vi "Merge_Raw_DF_metadata.vi"(4 "New Values In":string[](array[string]), 5 "New Chs In":string[](array[string]), 6 "Orig Values In":string[][](array[string]), 7 "Orig Chs In":string[](array[string])) -> (0 "Channel Values Out":string[][](array[string]), 1 "Ch names Out":string[](array[string]), 3 "Original values":string[](array[string]))   [LabVIEW 2020]
panel:
  out "Case":string
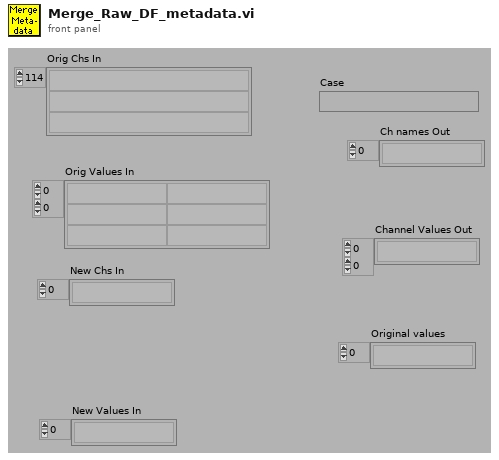
[diagram p1: front panel]
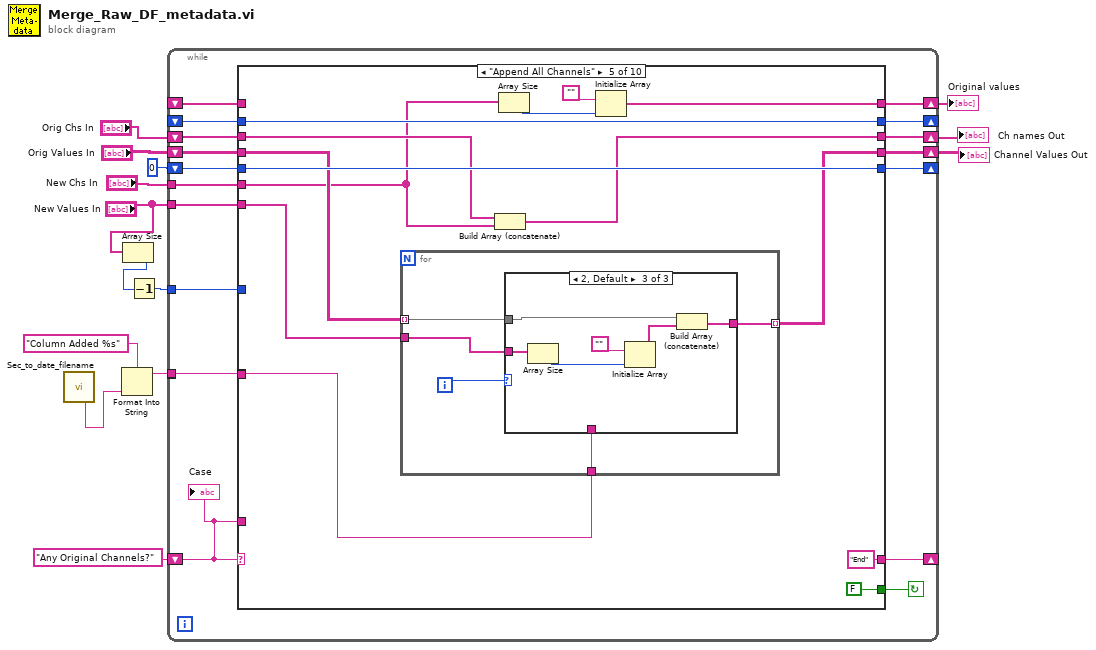
[diagram p0: block diagram]
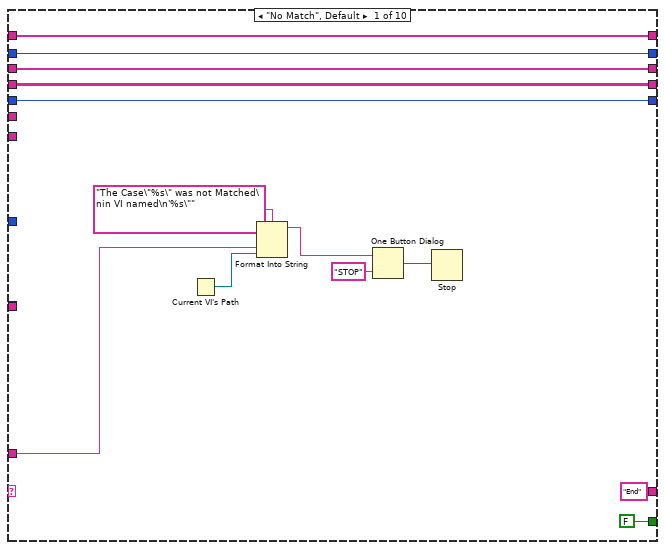
[diagram p2: hidden frame]
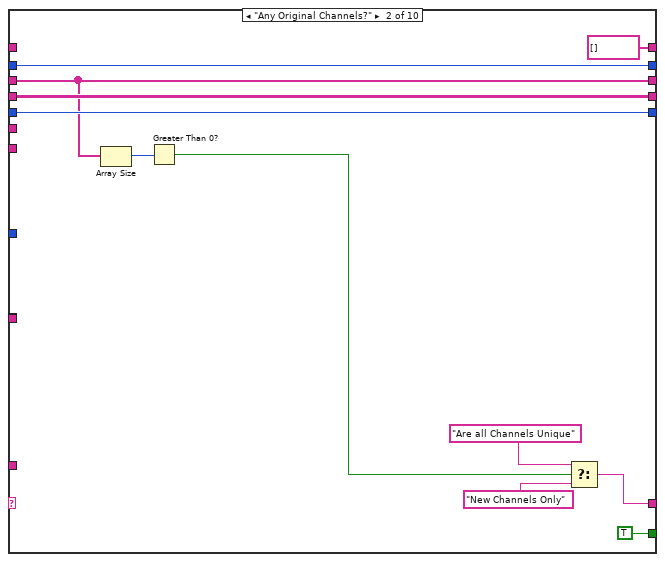
[diagram p3: hidden frame]
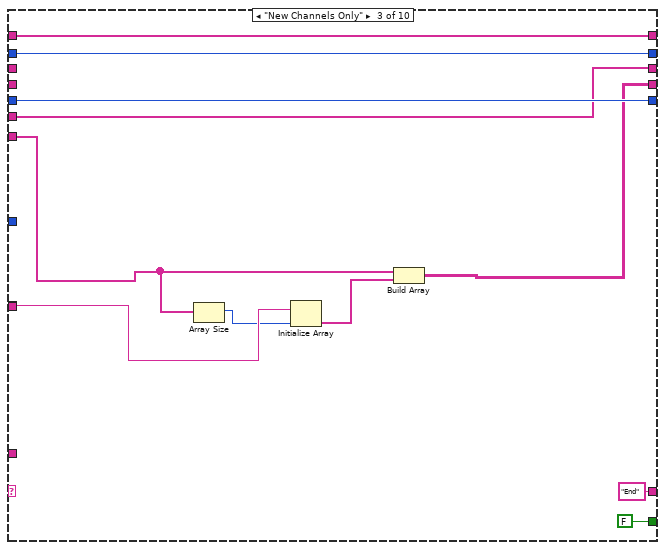
[diagram p4: hidden frame]
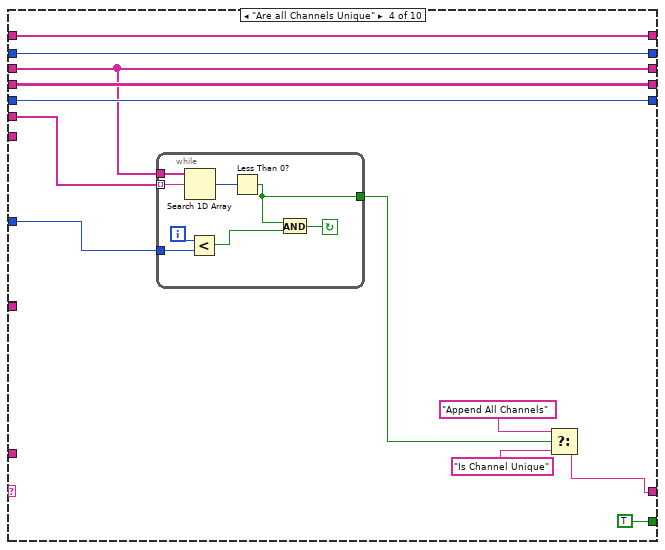
[diagram p5: hidden frame]
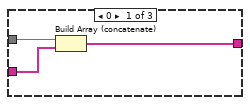
[diagram p6: hidden frame]
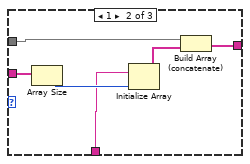
[diagram p7: hidden frame]
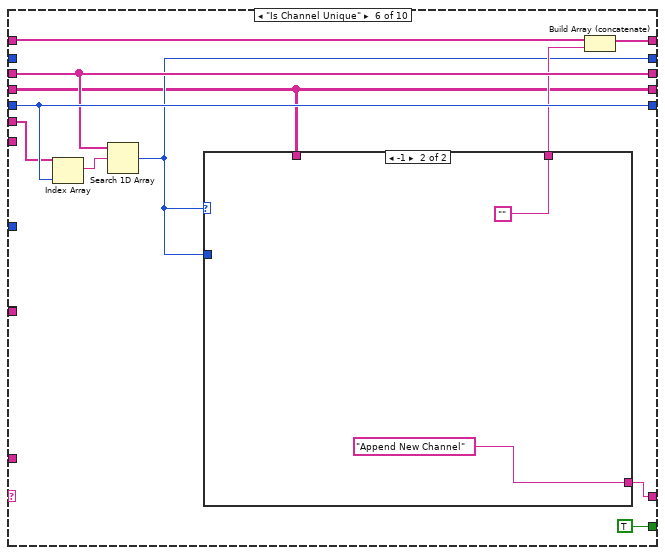
[diagram p8: hidden frame]
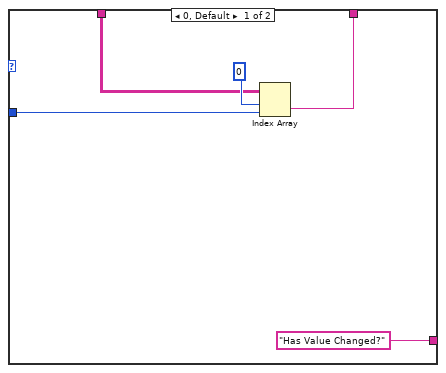
[diagram p9: hidden frame]
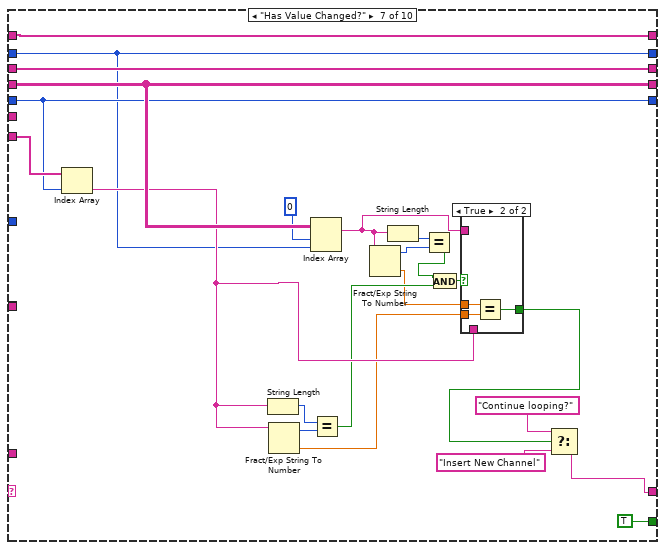
[diagram p10: hidden frame]
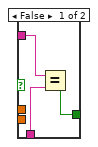
[diagram p11: hidden frame]
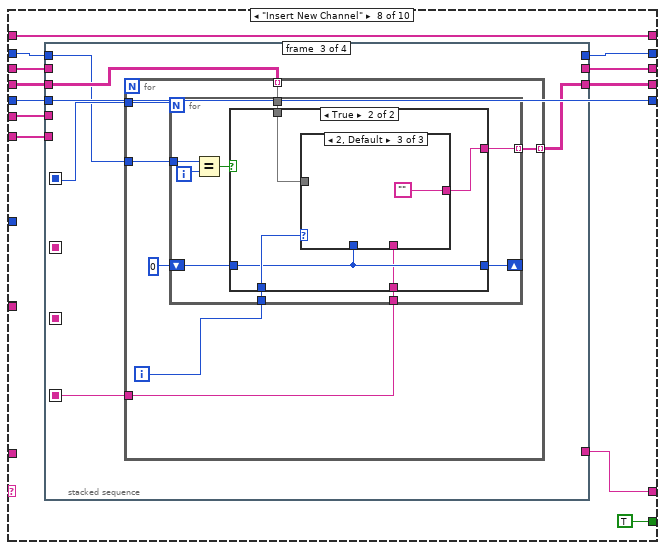
[diagram p12: hidden frame]
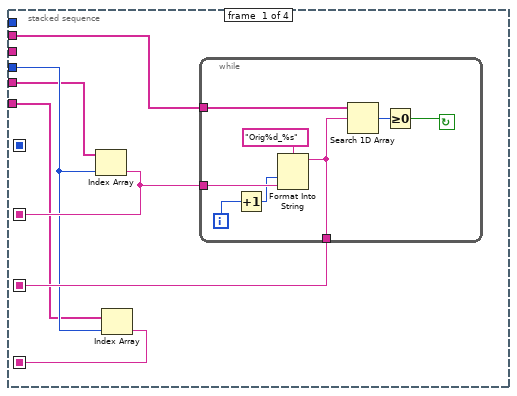
[diagram p13: hidden frame]
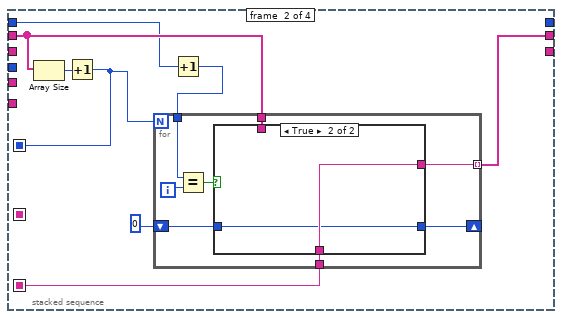
[diagram p14: hidden frame]
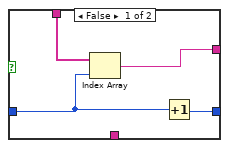
[diagram p15: hidden frame]
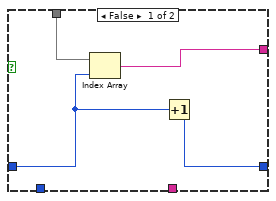
[diagram p16: hidden frame]
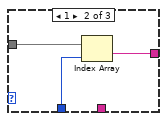
[diagram p18: hidden frame]
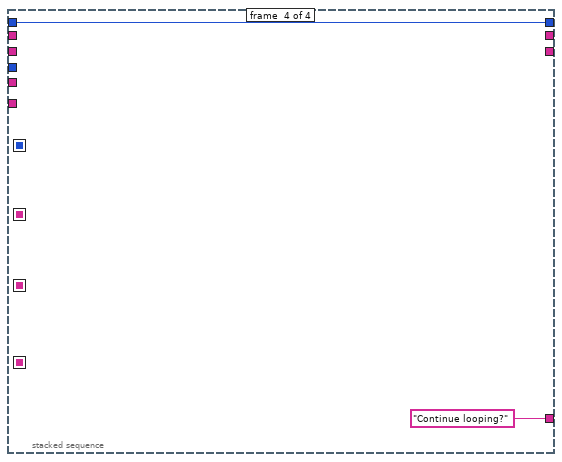
[diagram p19: hidden frame]
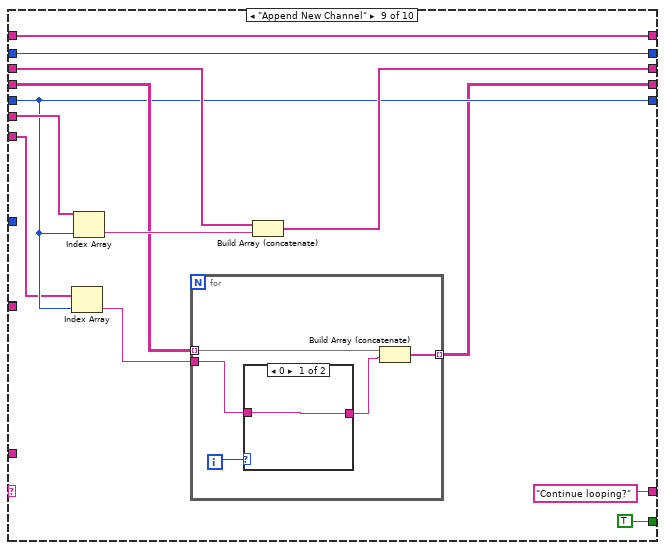
[diagram p20: hidden frame]
diagram:
  n1 = call "Sec_to_date_filename.vi"() -> ("YYYY-mm-DD HH:MM"=w1:string)  [unwired: 6 in, 9 out]
  n2 = Format Into String(format string="Column Added %s" ("Format String"), w1) -> (resulting string=w4:string)  [unwired: 2 in, 1 out]
  n3 = Array Size(array="New Values In") -> (size(s)=w10:i32)
  n4 = Decrement(x=w10) -> (x-1=w9:i32)
  n5 = while {
    tunnel: w4 -> [w17]
    tunnel: w4 -> [w18]
    shift-left: _ -> [w20]
    shift-right: [w19] -> _
    tunnel: "New Values In" -> [w21]
    tunnel: "New Chs In" -> [w22]
    tunnel: w9 -> [w23]
    shift-left: 0 -> [w24]
    shift-right: [w25] -> _
    shift-left: "Orig Values In" -> [w27]
    shift-right: [w26] -> w12
    shift-left: "Orig Chs In" -> [w28]
    shift-right: [w29] -> w13
    shift-left: "Any Original Channels?" -> [w31]
    shift-right: [w30] -> _
    shift-right: [w15] -> w2
    shift-left: _ -> [w16]
    stop <- w32 continue-if-true
    n6 = case shown="\"Append All Channels\"" w31 {
      tunnel: [FALSE ("Results File?") TRUE ("Results File?") FALSE ("Results File?") TRUE ("Results File?") FALSE ("Results File?") TRUE ("Results File?") TRUE ("Results File?") TRUE ("Results File?") TRUE ("Results File?") w280] -> w32
      tunnel: w31 -> [w40 _ _ _ _ _ _ _ _ _]
      tunnel: w22 -> [_ _ w62 w72 w89 w127 _ w177 w266 _]
      tunnel: w21 -> [_ _ w61 _ w95 _ w159 w176 w260 _]
      tunnel: ["End" w51 "End" ("f") w78 "End" ("f") w131 w160 w172 "Continue looping?" "Is Channel Unique"] -> w30
      tunnel: [w37 w49 w62 w73 w97 w128 w162 w173 w263 w282] -> w29
      tunnel: w28 -> [w37 w49 _ w73 w98 w128 w162 w179 w264 w282]
      tunnel: w27 -> [w36 w55 _ w77 w96 w122 w158 w174 w262 w283]
      tunnel: [w36 w55 w63 w77 w94 w122 w158 w175 w258 w283] -> w26
      tunnel: [w35 w54 w66 w76 w100 w130 w150 w178 w261 w277] -> w25
      tunnel: w24 -> [w35 w54 w66 w76 w100 w130 w150 w178 w261 w278]
      tunnel: w23 -> [_ _ _ w71 _ _ _ _ _ w281]
      tunnel: w20 -> [w34 w53 w65 w69 w93 _ w149 w171 w256 w276]
      tunnel: [w34 w53 w65 w69 w93 w123 w149 w170 w256 w276] -> w19
      tunnel: w18 -> [_ _ w60 _ w92 _ _ _ _ _]
      tunnel: w17 -> [_ _ _ _ _ _ _ _ _ _]
      tunnel: w16 -> [w33 _ w57 w68 _ w125 w140 w169 w255 w275]
      tunnel: [w33 string[] [] w57 w68 w88 w124 w140 w169 w255 w275] -> w15
      frame "No Match", Default {
        n7 = Current VI's Path() -> (path=w41:path)
        n8 = Format Into String(format string="The Case\"%s\" was not Matched\nin VI named\n'%s\"" ("Format String"), w40, w41) -> (resulting string=w44:string)  [unwired: 2 in, 1 out]
        n9 = One Button Dialog(message=w44, button name ("OK")="STOP") -> (true=w42:bool)
        n10 = Stop(stop? (T)=w42) -> ()
      }
      frame "Any Original Channels?" {
        n11 = Array Size(array=w49) -> (size(s)=w48:i32)
        n12 = Greater Than 0?(x=w48) -> (x > 0?=w47:bool)
        n13 = Select(t="Are all Channels Unique", s=w47, f="New Channels Only") -> (s? t:f=w51:string)
      }
      frame "New Channels Only" {
        n14 = Array Size(array=w61) -> (size(s)=w59:i32)
        n15 = Initialize Array(w60, w59) -> (w58:string[])
        n16 = Build Array(w61, w58) -> (w63:string[][])
      }
      frame "Are all Channels Unique" {
        n17 = while {
          tunnel: [w80] -> w70
          tunnel: w71 -> [w83]
          tunnel: w72 -> [w86] mode=indexing
          tunnel: w73 -> [w87]
          i -> [w84]
          stop <- w81 continue-if-true
          n18 = Search 1D Array(1D array=w87, element=w86) -> (index of element=w85:i32)  [unwired: 1 in]
          n19 = Less?(x=w84, y=w83) -> (x < y?=w82:bool)
          n20 = Less Than 0?(x=w85) -> (x < 0?=w80:bool)
          n21 = And(x=w80, y=w82) -> (x .and. y?=w81:bool)
        }
        n22 = Select(t="Append All Channels" ("f"), s=w70, f="Is Channel Unique") -> (s? t:f=w78:string)
      }
      frame "Append All Channels" {
        n23 = for {
          tunnel: w96 -> [w106] mode=indexing
          tunnel: w95 -> [w105]
          tunnel: [w104] -> w94 mode=indexing
          tunnel: w92 -> [w103]
          i -> [w102]
          n24 = case shown="2, Default" w102 {
            tunnel: w106 -> [w109 w111 w118]
            tunnel: w105 -> [w108 w115 w121]
            tunnel: [w107 w110 w117] -> w104
            tunnel: w103 -> [_ w113 _]
            frame 0 {
              n25 = Build Array (concatenate)(w109, w108) -> (w107:string[])
            }
            frame 1 {
              n26 = Array Size(array=w115) -> (size(s)=w114:i32)
              n27 = Initialize Array(w113, w114) -> (w112:string[])
              n28 = Build Array (concatenate)(w111, w112) -> (w110:string[])
            }
            frame 2, Default {
              n29 = Array Size(array=w121) -> (size(s)=w120:i32)
              n30 = Initialize Array("", w120) -> (w119:string[])
              n31 = Build Array (concatenate)(w118, w119) -> (w117:string[])
            }
          }
        }
        n32 = Build Array (concatenate)(w98, w89) -> (w97:string[])
        n33 = Array Size(array=w89) -> (size(s)=w90:i32)
        n34 = Initialize Array("", w90) -> (w88:string[])
      }
      frame "Is Channel Unique" {
        n35 = Index Array(array=w127, index=w130) -> (element=w129:string)
        n36 = Search 1D Array(1D array=w128, element=w129) -> (index of element=w123:i32)  [unwired: 1 in]
        n37 = case shown="-1" w123 {
          tunnel: ["Has Value Changed?" ("f") "Append New Channel"] -> w131
          tunnel: [w135 ""] -> w126
          tunnel: w123 -> [w136 _]
          tunnel: w122 -> [w134 _]
          frame 0, Default {
            n38 = Index Array(array=w134, index (row)=0, index (col)=w136) -> (element=w135:string)
          }
          frame -1 {
          }
        }
        n39 = Build Array (concatenate)(w125, w126) -> (w124:string[])
      }
      frame "Has Value Changed?" {
        n40 = Index Array(array=w159, index=w150) -> (element=w153:string)
        n41 = String Length(string=w153) -> (length=w155:i32)
        n42 = Fract/Exp String To Number(string=w153) -> (offset past number=w154:i32, number=w151:dbl)  [unwired: 3 in]
        n43 = Index Array(array=w158, index (row)=0, index (col)=w149) -> (element=w143:string)
        n44 = Equal?(x=w155, y=w154) -> (x = y?=w152:bool)
        n45 = Fract/Exp String To Number(string=w143) -> (offset past number=w147:i32, number=w144:dbl)  [unwired: 3 in]
        n46 = String Length(string=w143) -> (length=w148:i32)
        n47 = Equal?(x=w148, y=w147) -> (x = y?=w146:bool)
        n48 = And(x=w146, y=w152) -> (x .and. y?=w145:bool)
        n49 = case shown="True" w145 {
          tunnel: w144 -> [_ w168]
          tunnel: w151 -> [_ w167]
          tunnel: [w163 w166] -> w141
          tunnel: w143 -> [w165 _]
          tunnel: w153 -> [w164 _]
          frame False {
            n50 = Equal?(x=w165, y=w164) -> (x = y?=w163:bool)
          }
          frame True {
            n51 = Equal?(x=w168, y=w167) -> (x = y?=w166:bool)
          }
        }
        n52 = Select(t="Continue looping?", s=w141, f="Insert New Channel") -> (s? t:f=w160:string)
      }
      frame "Insert New Channel" {
        n53 = stacked-sequence {
          seq-local: [w186 _ _ _] -> [_ _ _ _]
          seq-local: [w185 _ _ _] -> [_ w198 _ _]
          seq-local: [w182 _ _ _] -> [_ _ w221 _]
          seq-local: [_ w200 _ _] -> [_ _ w219 _]
          tunnel: w179 -> [w187 w201 _ _]
          tunnel: w178 -> [w184 _ _ _]
          tunnel: w177 -> [w181 _ _ _]
          tunnel: w176 -> [w183 _ _ _]
          tunnel: [_ _ w222 _] -> w175
          tunnel: w174 -> [_ _ w220 _]
          tunnel: [_ w199 _ _] -> w173
          tunnel: [_ _ _ "Continue looping?"] -> w172
          tunnel: w171 -> [_ w197 w218 w253]
          tunnel: [_ _ _ w253] -> w170
          frame #0 {
            n54 = Index Array(array=w181, index=w184) -> (element=w186:string)
            n55 = Index Array(array=w183, index=w184) -> (element=w182:string)
            n56 = while {
              tunnel: [w188] -> w185
              tunnel: w186 -> [w194]
              tunnel: w187 -> [w195]
              i -> [w190]
              stop <- w191 continue-if-true
              n57 = Increment(x=w190) -> (x+1=w189:i32)
              n58 = Format Into String(format string="Orig%d_%s" ("Format String"), w189, w194) -> (resulting string=w188:string)  [unwired: 2 in, 1 out]
              n59 = Search 1D Array(1D array=w195, element=w188) -> (index of element=w192:i32)  [unwired: 1 in]
              n60 = Greater Or Equal To 0?(x=w192) -> (x >= 0?=w191:bool)
            }
          }
          frame #1 {
            n61 = Array Size(array=w201) -> (size(s)=w203:i32)
            n62 = Increment(x=w203) -> (x+1=w200:i32)
            n63 = Increment(x=w197) -> (x+1=w196:i32)
            n64 = for {
              N: w200 -> [_]
              shift-right: [w206] -> _
              shift-left: 0 -> [w207]
              tunnel: [w209] -> w199 mode=indexing
              tunnel: w198 -> [w208]
              tunnel: w201 -> [w205]
              tunnel: w196 -> [w204]
              i -> [w211]
              n65 = Equal?(x=w204, y=w211) -> (x = y?=w210:bool)
              n66 = case shown="True" w210 {
                tunnel: [w214 w217] -> w209
                tunnel: w208 -> [_ w217]
                tunnel: w205 -> [w215 _]
                tunnel: w207 -> [w213 w216]
                tunnel: [w212 w216] -> w206
                frame False {
                  n67 = Index Array(array=w215, index=w213) -> (element=w214:string)
                  n68 = Increment(x=w213) -> (x+1=w212:i32)
                }
                frame True {
                }
              }
            }
          }
          frame #2 {
            n69 = for {
              tunnel: w219 -> [w228]
              tunnel: w218 -> [w227]
              tunnel: [w226] -> w222 mode=indexing
              tunnel: w221 -> [w224]
              tunnel: w220 -> [w225] mode=indexing
              i -> [w223]
              n70 = for {
                N: w228 -> [_]
                shift-right: [w232] -> _
                shift-left: 0 -> [w233]
                tunnel: w227 -> [w237]
                tunnel: [w235] -> w226 mode=indexing
                tunnel: w225 -> [w234]
                tunnel: w223 -> [w231]
                tunnel: w224 -> [w230]
                i -> [w238]
                n71 = Equal?(x=w237, y=w238) -> (x = y?=w236:bool)
                n72 = case shown="True" w236 {
                  tunnel: [w241 w244] -> w235
                  tunnel: w234 -> [w242 w245]
                  tunnel: w233 -> [w240 w246]
                  tunnel: [w239 w246] -> w232
                  tunnel: w231 -> [_ w247]
                  tunnel: w230 -> [_ w243]
                  frame False {
                    n73 = Index Array(array=w242, index=w240) -> (element=w241:string)
                    n74 = Increment(x=w240) -> (x+1=w239:i32)
                  }
                  frame True {
                    n75 = case shown="2, Default" w247 {
                      tunnel: w246 -> [_ w251 _]
                      tunnel: w245 -> [_ w250 _]
                      tunnel: [w248 w249 ""] -> w244
                      tunnel: w243 -> [w248 _ _]
                      frame 0 {
                      }
                      frame 1 {
                        n76 = Index Array(array=w250, index=w251) -> (element=w249:string)
                      }
                      frame 2, Default {
                      }
                    }
                  }
                }
              }
            }
          }
          frame #3 {
          }
        }
      }
      frame "Append New Channel" {
        n77 = Index Array(array=w260, index=w261) -> (element=w259:string)
        n78 = Index Array(array=w266, index=w261) -> (element=w265:string)
        n79 = for {
          tunnel: w262 -> [w272] mode=indexing
          tunnel: w259 -> [w268]
          tunnel: [w271] -> w258 mode=indexing
          i -> [w270]
          n80 = case shown="0" w270 {
            tunnel: [w273 ""] -> w269
            tunnel: w268 -> [w273 _]
            frame 0 {
            }
            frame 1, Default {
            }
          }
          n81 = Build Array (concatenate)(w272, w269) -> (w271:string[])
        }
        n82 = Build Array (concatenate)(w264, w265) -> (w263:string[])
      }
      frame "Continue looping?" {
        n83 = Less?(x=w278, y=w281) -> (x < y?=w280:bool)
        n84 = Increment(x=w278) -> (x+1=w277:i32)
      }
    }
    "Case" <- w31
  }
  "Channel Values Out" <- w12
  "Ch names Out" <- w13
  "Original values" <- w2
